vi "Serialize Core.vi"(8 "error in (no error)":errorcluster, 11 "Serializable Message in":refnum<class "Serializable Msg.lvclass">) -> (0 "error out":errorcluster, 2 "Serialized Message":string)   [LabVIEW 2020, in "Serializer.lvlib" / "Serializable Message.lvlib" / "Serializable Msg.lvclass"]
uses:
  Serializable Msg.lvclass
  Serializable Msg.lvclass/Serializable Msg.ctl
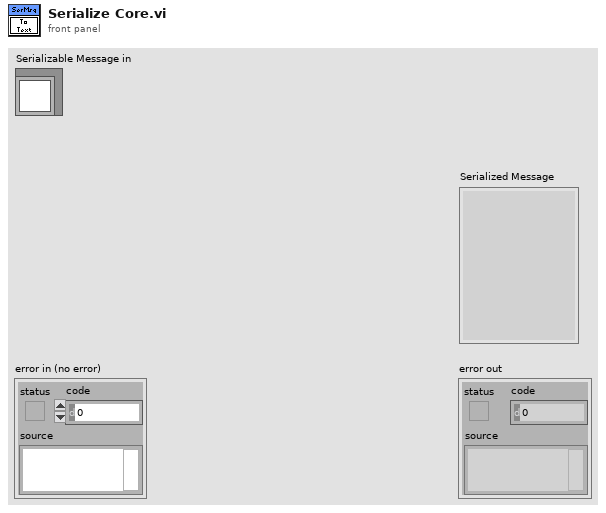
[diagram p1: front panel]
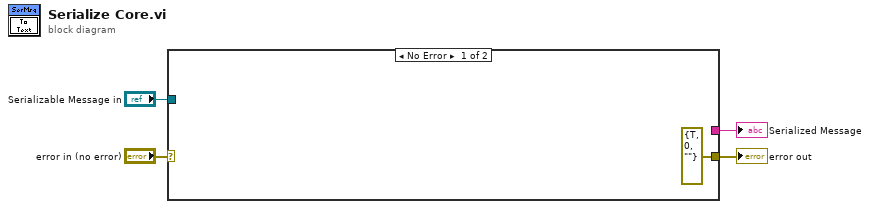
[diagram p0: block diagram]
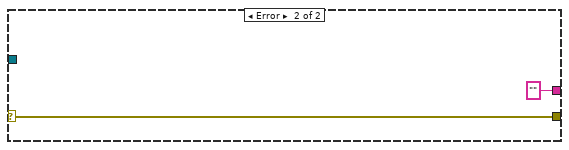
[diagram p2: hidden frame]
diagram:
  n1 = case shown="No Error" "error in (no error)" {
    selector: "error in (no error)" -> [_ w7]
    tunnel: "Serializable Message in" -> [_ _]
    tunnel: [_ "" ("<JSON>")] -> w3
    tunnel: [errorcluster {"status"=TRUE, "code"=0, "source"=""} ("error IO") w7] -> w2
    frame No Error {
    }
    frame Error {
    }
  }
  "error out" <- w2
  "Serialized Message" <- w3
